vi "MakeCursor.vi"(8 "WindowLoc":cluster{"r":i16, "c":i16}, 9 "Size":u8, 10 "Color":u32(colorbox), 11 "PicIn":picture) -> (3 "CursorOut":picture)   [LabVIEW 2014]
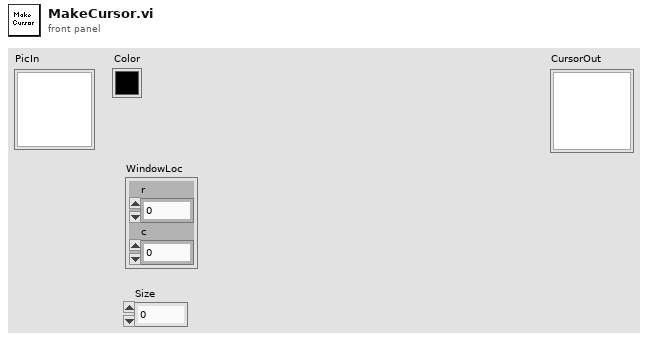
[diagram p1: front panel]
types:
  T1 = cluster{"left":i16, "top":i16, "right":i16, "bottom":i16}
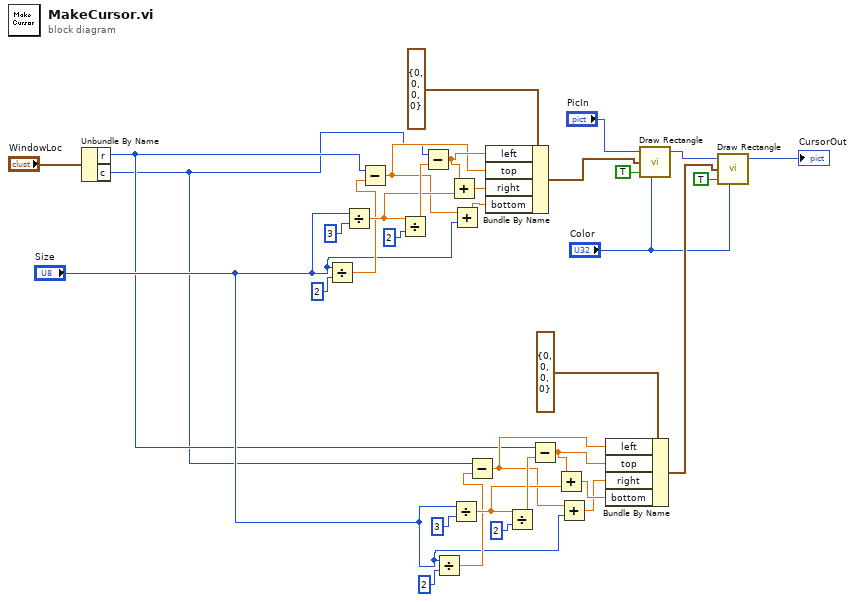
[diagram p0: block diagram]
diagram:
  n1 = Unbundle By Name("WindowLoc") -> ("r"=w3:i16, "c"=w2:i16)
  n2 = Divide(x="Size", y=u8 2) -> (x/y=w24:dbl)
  n3 = Divide(x="Size", y=u8 3) -> (x/y=w26:dbl)
  n4 = Subtract(x=w3, y=w24) -> (x-y=w22:dbl)
  n5 = Divide(x=w26, y=u8 2) -> (x/y=w28:dbl)
  n6 = Subtract(x=w2, y=w28) -> (x-y=w27:dbl)
  n7 = Divide(x="Size", y=u8 2) -> (x/y=w15:dbl)
  n8 = Add(x=w27, y=w26) -> (x+y=w25:dbl)
  n9 = Divide(x="Size", y=u8 3) -> (x/y=w16:dbl)
  n10 = Add(x=w22, y="Size") -> (x+y=w23:dbl)
  n11 = Subtract(x=w2, y=w15) -> (x-y=w12:dbl)
  n12 = Bundle By Name(cluster=T1 {"left"=0, "top"=0, "right"=0, "bottom"=0} ("Rect"), "left"=w27, "top"=w22, "right"=w25, "bottom"=w23) -> (w5:T1)
  n13 = Divide(x=w16, y=u8 2) -> (x/y=w18:dbl)
  n14 = Subtract(x=w3, y=w18) -> (x-y=w13:dbl)
  n15 = Add(x=w13, y=w16) -> (x+y=w11:dbl)
  n16 = Add(x=w12, y="Size") -> (x+y=w10:dbl)
  n17 = Bundle By Name(cluster=T1 {"left"=0, "top"=0, "right"=0, "bottom"=0} ("Rect"), "left"=w12, "top"=w13, "right"=w10, "bottom"=w11) -> (w4:T1)
  n18 = call <vilib>:"Draw Rectangle.vi"("picture"="PicIn", "rect"=w5, "fill?(F)"=TRUE, "color(black)"="Color") -> ("new picture"=w7:picture)  [unwired: 5 in]
  n19 = call <vilib>:"Draw Rectangle.vi"("picture"=w7, "rect"=w4, "fill?(F)"=TRUE, "color(black)"="Color") -> ("new picture"=→"CursorOut":picture)  [unwired: 5 in]
